vi "Potenza_celle.vi"() -> ()   [LabVIEW 2014]
uses:
  <vilib>/DAQmx/read.llb/DAQmx Read (Analog 2D DBL NChan NSamp).vi
  <vilib>/Analysis/baseanly.llb/Mean (DBL).vi
  <vilib>/DAQmx/create/channels.llb/DAQmx Create Channel (AI-Voltage-Basic).vi
  <vilib>/DAQmx/configure/timing.llb/DAQmx Timing (Sample Clock).vi
  <vilib>/DAQmx/miscellaneous.llb/DAQmx Fill In Error Info.vi
  <vilib>/Utility/file.llb/Write To Spreadsheet File (DBL).vi
  <vilib>/Analysis/NI_AALBase.lvlib
panel:
  in  "EXIT PROGRAM":bool
  in  "Resistenza":dbl=2.7 max=100000.0
  out "V_in(Volt)":dbl=0.2081706318888552 format="%.3f"
  out "Corrente (mA)":dbl=31.30588570078624 format="%.4f"
  in  "Fondo Scala AI1":dbl(ring)=5.0 items=["10"=10.0, "5"=5.0, "0.5"=0.5, "0.05"=0.05]
  in  "Fondo Scala AI0":dbl(ring)=0.5 items=["10"=10.0, "5"=5.0, "0.5"=0.5, "0.05"=0.05]
  in  "SALVA":bool=TRUE caption="ON\nOFF"
  out "power":cluster{dbl[], dbl[]}(graph)={[0.09478601789846895, 0.09478601789846895, 0.09519039454598441, 0.09519039454598441, 0.3692276546350666, 0.4111200013938477, 0.4111200013938477, 0.4208531577637632, 0.4208531577637632, 0.4255494982926404, 0.4402842388163407, 0.4435502862815671, 0.4435502862815671, 0.44368850953661537, 0.4491531483812087, 0.4513869200218114, 0.4513869200218114, 0.45480397968233355, 0.45480397968233355, 0.45705907451385963, 0.4584212187749075, 0.4605463340716431, 0.4605463340716431, 0.46217820728083553, 0.46357193005389463, 0.46446569248379926, 0.46484304010372907, 0.46543718331130957, 0.46615517263540734, 0.4390290005440171, 0.4390290005440171, 0.43334036436093054, 0.43334036436093054, 0.42420559561340954, 0.42420559561340954, 0.4270359081737125, 0.4270359081737125, 0.09544674857174822, 0.37267076173351704, 0.3881547056875887, 0.3881547056875887, 0.34106855480092135, 0.34106855480092135, 0.33109283770712306, 0.2068409232584436, 0.10409528201129736, 0.13447294260520917, 0.2984566947389119, 0.2984566947389119, 0.3700736078553747, 0.30440398953826114, 0.28259027086581395, 0.28259027086581395, 0.20417926683366502, 0.11794074102482587, 0.09686599380581434, 0.09553963187698407, 0.14140615930871372, 0.1509254439913714, 0.17778242825196688, 0.21380625131901929, 0.23492205647612335, 0.23492205647612335, 0.2729712800826533, 0.0, 0.0, 0.0, 0.0, 0.0, 0.0, 0.0, 0.0, 0.0, 0.0, 0.0, 0.0, 0.0, 0.0, 0.0, 0.0, 0.0, 0.0, 0.0, 0.0, 0.0, 0.0, 0.0, 0.0, 0.0, 0.0, 0.0, 0.0, 0.0, 0.0, 0.0, 0.0, 0.0, 0.0, 0.0, 0.0, 0.0, 0.0, 0.0, 0.0, 0.0, 0.0, 0.0, 0.0, 0.0, 0.0, 0.0, 0.0, 0.0, 0.0, 0.0, 0.0, 0.0, 0.0, 0.0, 0.0, 0.0, 0.0, 0.0, 0.0, 0.0, 0.0, 0.0, 0.0, 0.0, 0.0, 0.0, 0.0, 0.0, 0.0, 0.0, 0.0, 0.0, 0.0, 0.0, 0.0, 0.0, 0.0, 0.0, 0.0, 0.0, 0.0, 0.0, 0.0, 0.0, 0.0, 0.0, 0.0, 0.0, 0.0, 0.0, 0.0, 0.0, 0.0, 0.0, 0.0, 0.0, 0.0, 0.0, 0.0, 0.0, 0.0, 0.0, 0.0, 0.0, 0.0, 0.0, 0.0, 0.0, 0.0, 0.0, 0.0, 0.0, 0.0, 0.0, 0.0, 0.0, 0.0, 0.0, 0.0, 0.0, 0.0, 0.0, 0.0, 0.0, 0.0, 0.0, 0.0, 0.0, 0.0, 0.0, 0.0, 0.0, 0.0, 0.0, 0.0], [3.0170134735409397, 3.0170134735409397, 3.0201788565517984, 3.0201788565517984, 9.14140352368766, 7.85175000034162, 7.85175000034162, 7.221469220246045, 7.221469220246045, 6.8646837395680755, 5.412997641292046, 5.0489168328723055, 5.0489168328723055, 5.051448234534376, 4.348133054214019, 4.029529214267265, 4.029529214267265, 3.5183173733443494, 3.5183173733443494, 3.171630872751192, 2.9635146740029863, 2.588907716393703, 2.588907716393703, 2.2923528624342913, 2.0225602902113007, 1.8499819150481303, 1.7847675230358468, 1.6363589222375279, 1.534204978184801, 5.469082937412574, 5.469082937412574, 6.034056487177778, 6.034056487177778, 6.828298799638558, 6.828298799638558, 6.584690682350574, 6.584690682350574, 3.0455608576711226, 8.999642211687378, 8.636150436075797, 8.636150436075797, 9.145710007035497, 9.145710007035497, 9.095897977030202, 6.401982512490315, 3.325324661201692, 4.279414951081421, 8.728058986798336, 8.728058986798336, 9.110541910816105, 8.810402080562293, 8.426688585183642, 8.426688585183642, 6.40651230214226, 3.7818575624102304, 3.1124825241913823, 3.07055743646646, 4.5111823216029405, 4.79808672222816, 5.612649488498093, 6.681955401946596, 7.264660979738571, 7.264660979738571, 8.215200355082505, 0.0, 0.0, 0.0, 0.0, 0.0, 0.0, 0.0, 0.0, 0.0, 0.0, 0.0, 0.0, 0.0, 0.0, 0.0, 0.0, 0.0, 0.0, 0.0, 0.0, 0.0, 0.0, 0.0, 0.0, 0.0, 0.0, 0.0, 0.0, 0.0, 0.0, 0.0, 0.0, 0.0, 0.0, 0.0, 0.0, 0.0, 0.0, 0.0, 0.0, 0.0, 0.0, 0.0, 0.0, 0.0, 0.0, 0.0, 0.0, 0.0, 0.0, 0.0, 0.0, 0.0, 0.0, 0.0, 0.0, 0.0, 0.0, 0.0, 0.0, 0.0, 0.0, 0.0, 0.0, 0.0, 0.0, 0.0, 0.0, 0.0, 0.0, 0.0, 0.0, 0.0, 0.0, 0.0, 0.0, 0.0, 0.0, 0.0, 0.0, 0.0, 0.0, 0.0, 0.0, 0.0, 0.0, 0.0, 0.0, 0.0, 0.0, 0.0, 0.0, 0.0, 0.0, 0.0, 0.0, 0.0, 0.0, 0.0, 0.0, 0.0, 0.0, 0.0, 0.0, 0.0, 0.0, 0.0, 0.0, 0.0, 0.0, 0.0, 0.0, 0.0, 0.0, 0.0, 0.0, 0.0, 0.0, 0.0, 0.0, 0.0, 0.0, 0.0, 0.0, 0.0, 0.0, 0.0, 0.0, 0.0, 0.0, 0.0, 0.0, 0.0, 0.0, 0.0, 0.0]}
  out "Corrente":dbl[](array[numeric])=[31.82973122441588, 31.82973122441588, 31.727769077507247, 31.727769077507247, 24.758176720870885, 19.098438348222675, 19.098438348222675, 17.159118535828263, 17.159118535828263, 16.131340225073874, 12.294325265524694, 11.382963756373808, 11.382963756373808, 11.38512295441247, 9.680736002597579, 8.92699596628222, 8.92699596628222, 7.735898388140281, 7.735898388140281, 6.939214315183709, 6.464610608389228, 5.621383832339808, 5.621383832339808, 4.959889554120362, 4.3629912837392, 3.9830324284126934, 3.8395057450738177, 3.5157460145229575, 3.291189432718672, 12.457224763365586, 12.457224763365586, 13.92451980806476, 13.92451980806476, 16.096673099666933, 16.096673099666933, 15.41952457935226, 15.41952457935226, 31.90848198859017, 24.14904289734081, 22.249248326842938, 22.249248326842938, 26.814873075513415, 26.814873075513415, 27.472348964178497, 30.951237364625207, 31.945008428343538, 31.823613495579487, 29.24397120471226, 29.24397120471226, 24.618188699304703, 28.943122900348506, 29.81945754666479, 29.81945754666479, 31.37689933699946, 32.06574360605527, 32.13183906863047, 32.13909637437248, 31.902304281910812, 31.79110556403248, 31.57032752721442, 31.252385562742422, 30.923707585017354, 30.923707585017354, 30.095475071938026] format="%#_3f"
  out "Tensione":dbl[](array[numeric])=[0.09478601789846895, 0.09478601789846895, 0.09519039454598441, 0.09519039454598441, 0.3692276546350666, 0.4111200013938477, 0.4111200013938477, 0.4208531577637632, 0.4208531577637632, 0.4255494982926404, 0.4402842388163407, 0.4435502862815671, 0.4435502862815671, 0.44368850953661537, 0.4491531483812087, 0.4513869200218114, 0.4513869200218114, 0.45480397968233355, 0.45480397968233355, 0.45705907451385963, 0.4584212187749075, 0.4605463340716431, 0.4605463340716431, 0.46217820728083553, 0.46357193005389463, 0.46446569248379926, 0.46484304010372907, 0.46543718331130957, 0.46615517263540734, 0.4390290005440171, 0.4390290005440171, 0.43334036436093054, 0.43334036436093054, 0.42420559561340954, 0.42420559561340954, 0.4270359081737125, 0.4270359081737125, 0.09544674857174822, 0.37267076173351704, 0.3881547056875887, 0.3881547056875887, 0.34106855480092135, 0.34106855480092135, 0.33109283770712306, 0.2068409232584436, 0.10409528201129736, 0.13447294260520917, 0.2984566947389119, 0.2984566947389119, 0.3700736078553747, 0.30440398953826114, 0.28259027086581395, 0.28259027086581395, 0.20417926683366502, 0.11794074102482587, 0.09686599380581434, 0.09553963187698407, 0.14140615930871372, 0.1509254439913714, 0.17778242825196688, 0.21380625131901929, 0.23492205647612335, 0.23492205647612335, 0.2729712800826533] format="%#_3f"
  out "Potenza (mW)":dbl[](array[numeric])=[3.0170134735409397, 3.0170134735409397, 3.0201788565517984, 3.0201788565517984, 9.14140352368766, 7.85175000034162, 7.85175000034162, 7.221469220246045, 7.221469220246045, 6.8646837395680755, 5.412997641292046, 5.0489168328723055, 5.0489168328723055, 5.051448234534376, 4.348133054214019, 4.029529214267265, 4.029529214267265, 3.5183173733443494, 3.5183173733443494, 3.171630872751192, 2.9635146740029863, 2.588907716393703, 2.588907716393703, 2.2923528624342913, 2.0225602902113007, 1.8499819150481303, 1.7847675230358468, 1.6363589222375279, 1.534204978184801, 5.469082937412574, 5.469082937412574, 6.034056487177778, 6.034056487177778, 6.828298799638558, 6.828298799638558, 6.584690682350574, 6.584690682350574, 3.0455608576711226, 8.999642211687378, 8.636150436075797, 8.636150436075797, 9.145710007035497, 9.145710007035497, 9.095897977030202, 6.401982512490315, 3.325324661201692, 4.279414951081421, 8.728058986798336, 8.728058986798336, 9.110541910816105, 8.810402080562293, 8.426688585183642, 8.426688585183642, 6.40651230214226, 3.7818575624102304, 3.1124825241913823, 3.07055743646646, 4.5111823216029405, 4.79808672222816, 5.612649488498093, 6.681955401946596, 7.264660979738571, 7.264660979738571, 8.215200355082505] format="%#_3f"
  out "Grafico Dati Acquisiti":cluster{dbl[], dbl[]}(graph)={[0.09478601789846895, 0.09478601789846895, 0.09519039454598441, 0.09519039454598441, 0.3692276546350666, 0.4111200013938477, 0.4111200013938477, 0.4208531577637632, 0.4208531577637632, 0.4255494982926404, 0.4402842388163407, 0.4435502862815671, 0.4435502862815671, 0.44368850953661537, 0.4491531483812087, 0.4513869200218114, 0.4513869200218114, 0.45480397968233355, 0.45480397968233355, 0.45705907451385963, 0.4584212187749075, 0.4605463340716431, 0.4605463340716431, 0.46217820728083553, 0.46357193005389463, 0.46446569248379926, 0.46484304010372907, 0.46543718331130957, 0.46615517263540734, 0.4390290005440171, 0.4390290005440171, 0.43334036436093054, 0.43334036436093054, 0.42420559561340954, 0.42420559561340954, 0.4270359081737125, 0.4270359081737125, 0.09544674857174822, 0.37267076173351704, 0.3881547056875887, 0.3881547056875887, 0.34106855480092135, 0.34106855480092135, 0.33109283770712306, 0.2068409232584436, 0.10409528201129736, 0.13447294260520917, 0.2984566947389119, 0.2984566947389119, 0.3700736078553747, 0.30440398953826114, 0.28259027086581395, 0.28259027086581395, 0.20417926683366502, 0.11794074102482587, 0.09686599380581434, 0.09553963187698407, 0.14140615930871372, 0.1509254439913714, 0.17778242825196688, 0.21380625131901929, 0.23492205647612335, 0.23492205647612335, 0.2729712800826533, 0.0, 0.0, 0.0, 0.0, 0.0, 0.0, 0.0, 0.0, 0.0, 0.0, 0.0, 0.0, 0.0, 0.0, 0.0, 0.0, 0.0, 0.0, 0.0, 0.0, 0.0, 0.0, 0.0, 0.0, 0.0, 0.0, 0.0, 0.0, 0.0, 0.0, 0.0, 0.0, 0.0, 0.0, 0.0, 0.0, 0.0, 0.0, 0.0, 0.0, 0.0, 0.0, 0.0, 0.0, 0.0, 0.0, 0.0, 0.0, 0.0, 0.0, 0.0, 0.0, 0.0, 0.0, 0.0, 0.0, 0.0, 0.0, 0.0, 0.0, 0.0, 0.0, 0.0, 0.0, 0.0, 0.0, 0.0, 0.0, 0.0, 0.0, 0.0, 0.0, 0.0, 0.0, 0.0, 0.0, 0.0, 0.0, 0.0, 0.0, 0.0, 0.0, 0.0, 0.0, 0.0, 0.0, 0.0, 0.0, 0.0, 0.0, 0.0, 0.0, 0.0, 0.0, 0.0, 0.0, 0.0, 0.0, 0.0, 0.0, 0.0, 0.0, 0.0, 0.0, 0.0, 0.0, 0.0, 0.0, 0.0, 0.0, 0.0, 0.0, 0.0, 0.0, 0.0, 0.0, 0.0, 0.0, 0.0, 0.0, 0.0, 0.0, 0.0, 0.0, 0.0, 0.0, 0.0, 0.0, 0.0, 0.0, 0.0, 0.0, 0.0, 0.0, 0.0, 0.0], [31.82973122441588, 31.82973122441588, 31.727769077507247, 31.727769077507247, 24.758176720870885, 19.098438348222675, 19.098438348222675, 17.159118535828263, 17.159118535828263, 16.131340225073874, 12.294325265524694, 11.382963756373808, 11.382963756373808, 11.38512295441247, 9.680736002597579, 8.92699596628222, 8.92699596628222, 7.735898388140281, 7.735898388140281, 6.939214315183709, 6.464610608389228, 5.621383832339808, 5.621383832339808, 4.959889554120362, 4.3629912837392, 3.9830324284126934, 3.8395057450738177, 3.5157460145229575, 3.291189432718672, 12.457224763365586, 12.457224763365586, 13.92451980806476, 13.92451980806476, 16.096673099666933, 16.096673099666933, 15.41952457935226, 15.41952457935226, 31.90848198859017, 24.14904289734081, 22.249248326842938, 22.249248326842938, 26.814873075513415, 26.814873075513415, 27.472348964178497, 30.951237364625207, 31.945008428343538, 31.823613495579487, 29.24397120471226, 29.24397120471226, 24.618188699304703, 28.943122900348506, 29.81945754666479, 29.81945754666479, 31.37689933699946, 32.06574360605527, 32.13183906863047, 32.13909637437248, 31.902304281910812, 31.79110556403248, 31.57032752721442, 31.252385562742422, 30.923707585017354, 30.923707585017354, 30.095475071938026, 0.0, 0.0, 0.0, 0.0, 0.0, 0.0, 0.0, 0.0, 0.0, 0.0, 0.0, 0.0, 0.0, 0.0, 0.0, 0.0, 0.0, 0.0, 0.0, 0.0, 0.0, 0.0, 0.0, 0.0, 0.0, 0.0, 0.0, 0.0, 0.0, 0.0, 0.0, 0.0, 0.0, 0.0, 0.0, 0.0, 0.0, 0.0, 0.0, 0.0, 0.0, 0.0, 0.0, 0.0, 0.0, 0.0, 0.0, 0.0, 0.0, 0.0, 0.0, 0.0, 0.0, 0.0, 0.0, 0.0, 0.0, 0.0, 0.0, 0.0, 0.0, 0.0, 0.0, 0.0, 0.0, 0.0, 0.0, 0.0, 0.0, 0.0, 0.0, 0.0, 0.0, 0.0, 0.0, 0.0, 0.0, 0.0, 0.0, 0.0, 0.0, 0.0, 0.0, 0.0, 0.0, 0.0, 0.0, 0.0, 0.0, 0.0, 0.0, 0.0, 0.0, 0.0, 0.0, 0.0, 0.0, 0.0, 0.0, 0.0, 0.0, 0.0, 0.0, 0.0, 0.0, 0.0, 0.0, 0.0, 0.0, 0.0, 0.0, 0.0, 0.0, 0.0, 0.0, 0.0, 0.0, 0.0, 0.0, 0.0, 0.0, 0.0, 0.0, 0.0, 0.0, 0.0, 0.0, 0.0, 0.0, 0.0, 0.0, 0.0, 0.0, 0.0, 0.0, 0.0]}
  out "Pronto per la misura":bool=TRUE
  in  "Esegui la misura":bool
  out "Misure fatte":u16=64
  # "Dati acquisiti"
  # "NO\nSI"
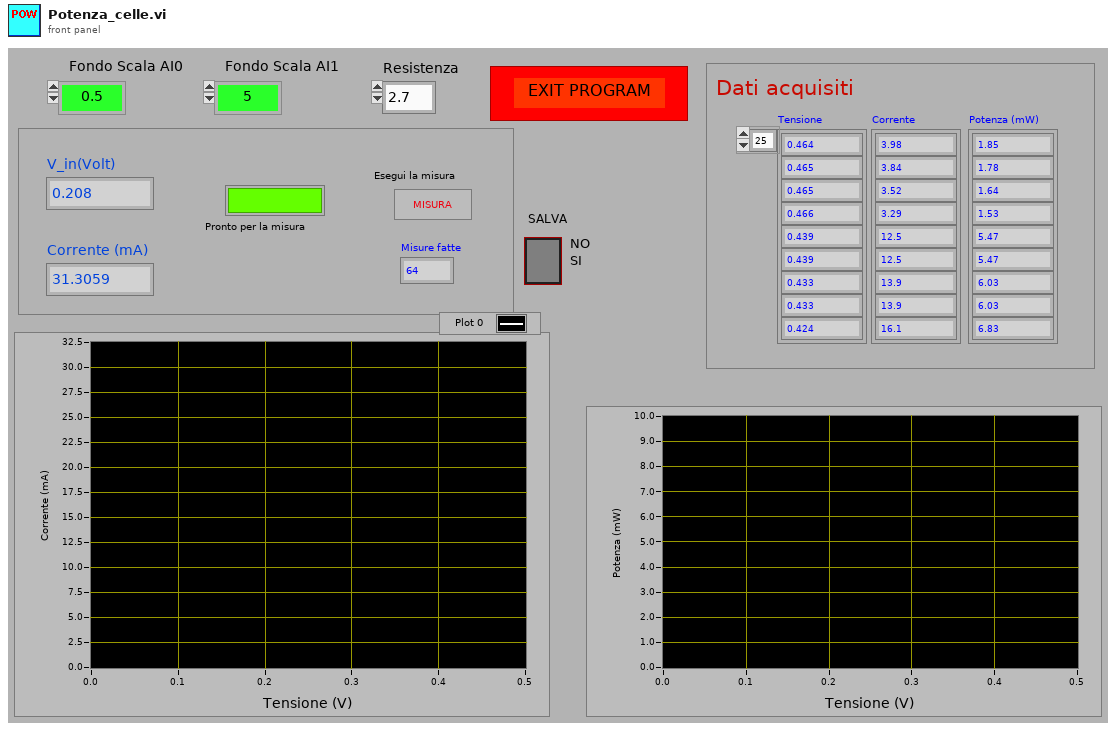
[diagram p1: front panel]
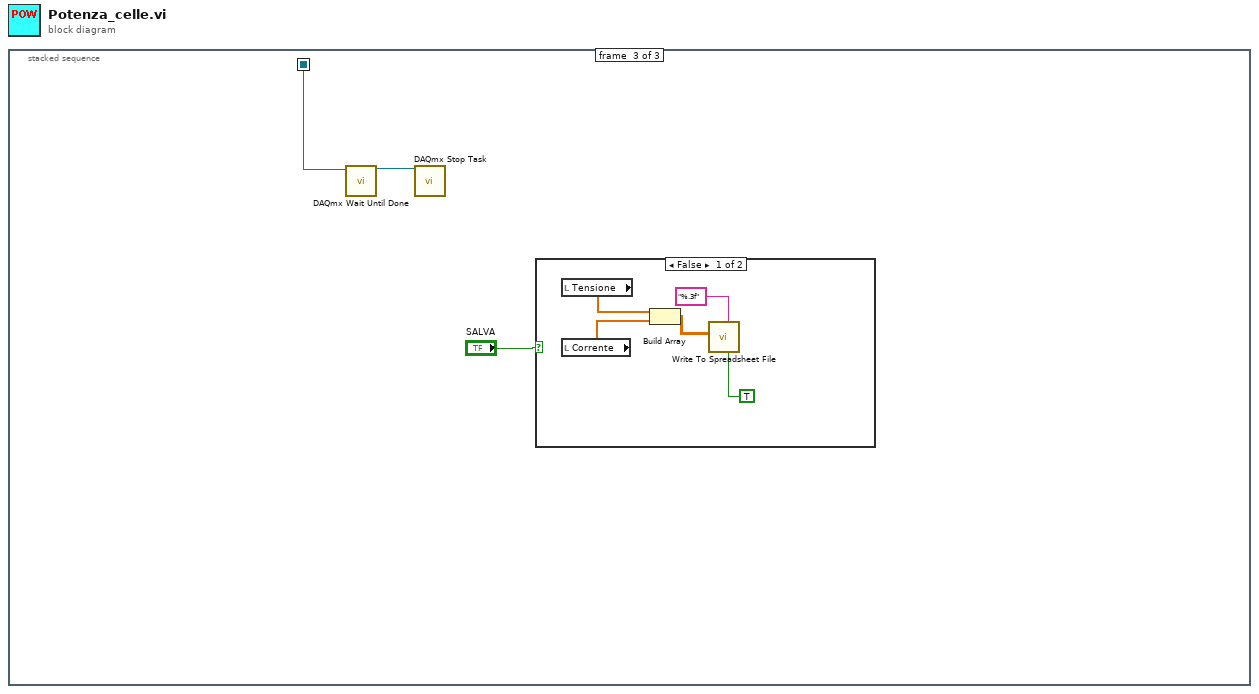
[diagram p0: block diagram]
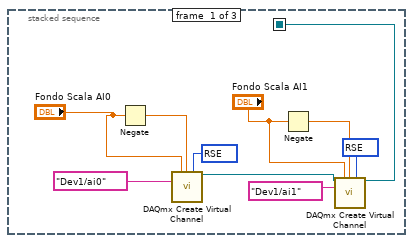
[diagram p2: hidden frame]
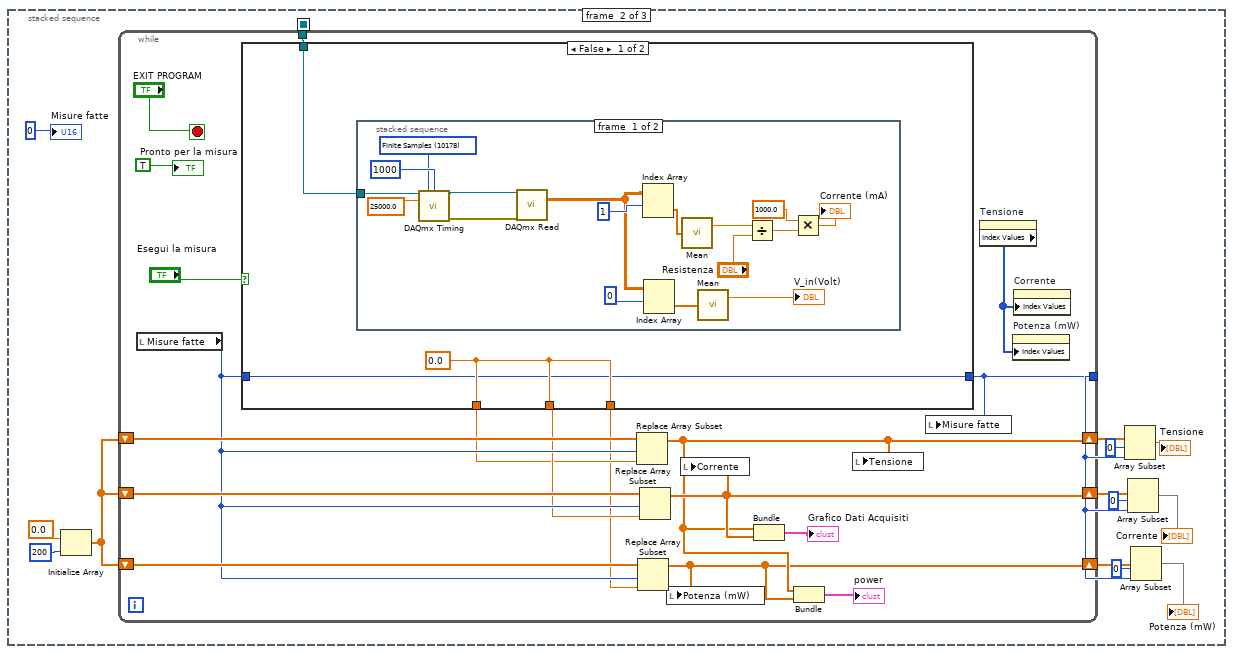
[diagram p3: hidden frame]
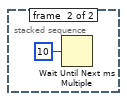
[diagram p4: hidden frame]
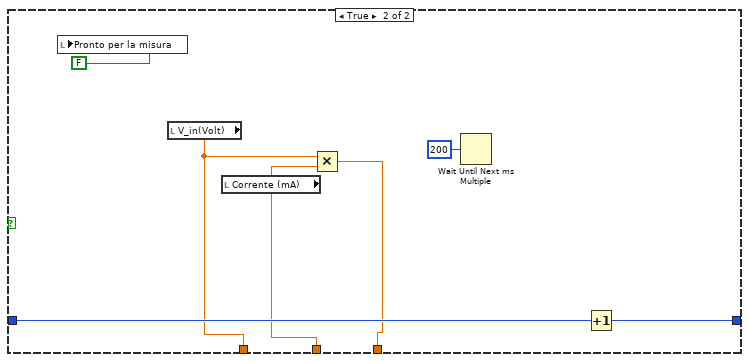
[diagram p5: hidden frame]
diagram:
  n1 = stacked-sequence {
    seq-local: [w1 _ _] -> [_ w11 w72]
    frame #0 {
      w6 = 10083 items=["default"=-1, "RSE"=10083, "NRSE"=10078, "Differential"=10106, "Pseudodifferential"=12529] ("input terminal configuration")
      w9 = 10083 items=["default"=-1, "RSE"=10083, "NRSE"=10078, "Differential"=10106, "Pseudodifferential"=12529] ("input terminal configuration")
      n2 = Negate(x="Fondo Scala AI0") -> (-x=w7:dbl)
      n3 = call-poly <vilib>:"DAQmx Create Virtual Channel.vi"("maximum value"="Fondo Scala AI0", "minimum value"=w7, "input terminal configuration"=w6, "physical channels"=tag "Dev1/ai0") -> ("task out"=w4:refnum<k21>)  [unwired: 5 in, 6 out]
      n4 = Negate(x="Fondo Scala AI1") -> (-x=w10:dbl)
      n5 = call-poly <vilib>:"DAQmx Create Virtual Channel.vi"("task in"=w4, "maximum value"="Fondo Scala AI1", "minimum value"=w10, "input terminal configuration"=w9, "physical channels"=tag "Dev1/ai1") -> ("task out"=w1:refnum<k21>)  [unwired: 4 in, 6 out]
    }
    frame #1 {
      n6 = Initialize Array(0.0 ("Element Data"), 200 ("Dimension Size")) -> (w22:dbl[])
      n7 = while {
        tunnel: [w41] -> w15
        shift-left: w22 -> [w38]
        shift-right: [w32] -> w18
        shift-left: w22 -> [w39]
        shift-right: [w30] -> w21
        shift-left: w22 -> [w40]
        shift-right: [w29] -> w16
        tunnel: w11 -> [w28]
        stop <- "EXIT PROGRAM" stop-if-true
        n8 = local read "Misure fatte"() -> (w37:u16)
        n9 = case shown="False" "Esegui la misura" {
          tunnel: w37 -> [w44 w71]
          tunnel: [w44 w65] -> w41
          tunnel: [w45 w68] -> w35
          tunnel: [w45 w67] -> w36
          tunnel: [w45 w66] -> w34
          tunnel: w28 -> [w46 _]
          frame False {
            w45 = 0.0
            n10 = stacked-sequence {
              tunnel: w46 -> [w58 _]
              frame #0 {
                w59 = 10178 items=["Finite Samples"=10178, "Continuous Samples"=10123, "Hardware Timed Single Point"=12522] ("sample mode")
                n11 = call-poly <vilib>:"DAQmx Timing.vi"("task/channels in"=w58, "sample mode"=w59, "samples per channel"=u32 1000, "rate"=25000.0) -> ("task out"=w63:refnum<k21>, "error out"=w62:errorcluster)  [unwired: 3 in, 7 out]
                n12 = call-poly <vilib>:"DAQmx Read.vi"("task/channels in"=w63, "error in"=w62) -> ("data"=w47:dbl[][])  [unwired: 1 in, 12 out]
                n13 = Index Array(array=w47, index (row)=1) -> (element=w55:dbl[])  [unwired: 1 in]
                n14 = Index Array(array=w47, index (row)=0) -> (element=w54:dbl[])  [unwired: 1 in]
                n15 = call-poly <vilib>:"Mean.vi"("X"=w55) -> ("mean"=w57:dbl)  [unwired: 1 out]
                n16 = call-poly <vilib>:"Mean.vi"("X"=w54) -> ("mean"=→"V_in(Volt)":dbl)  [unwired: 1 out]
                n17 = Divide(x=w57, y="Resistenza") -> (x/y=w51:dbl)
                n18 = Multiply(x=1000.0, y=w51) -> (x*y=→"Corrente (mA)":dbl)
              }
              frame #1 {
                n19 = Wait Until Next ms Multiple(millisecond multiple=u32 10) -> ()  [unwired: 1 out]
              }
            }
          }
          frame True {
            n20 = local write "Pronto per la misura"(FALSE ("Pronto per la misura")) -> ()
            n21 = local read "V_in(Volt)"() -> (w68:dbl)
            n22 = local read "Corrente (mA)"() -> (w67:dbl)
            n23 = Multiply(x=w68, y=w67) -> (x*y=w66:dbl)
            n24 = Wait Until Next ms Multiple(millisecond multiple=u32 200) -> ()  [unwired: 1 out]
            n25 = Increment(x=w71) -> (x+1=w65:u16)
          }
        }
        n26 = Replace Array Subset(array=w39, new element=w35, index=w37) -> (w30:dbl[])
        n27 = Replace Array Subset(array=w40, new element=w34, index=w37) -> (w29:dbl[])
        n28 = Replace Array Subset(array=w38, new element=w36, index=w37) -> (w32:dbl[])
        n29 = local write "Potenza (mW)"(w29) -> ()
        n30 = local write "Corrente"(w32) -> ()
        n31 = Bundle(w30, w32) -> (→"Grafico Dati Acquisiti":cluster{dbl[], dbl[]})  [unwired: 1 out]
        n32 = Bundle(w30, w29) -> (→"power":cluster{dbl[], dbl[]})  [unwired: 1 out]
        n33 = local write "Tensione"(w30) -> ()
        n34 = local write "Misure fatte"(w41) -> ()
        n35 = property on="Tensione" class="Arr (strict)"() -> ("Index Values"=w27:u32[])  [unwired: 2 in, 2 out]
        n36 = property on="Potenza (mW)" class="Arr (strict)"("Index Values"=w27) -> ()  [unwired: 2 in, 2 out]
        n37 = property on="Corrente" class="Arr (strict)"("Index Values"=w27) -> ()  [unwired: 2 in, 2 out]
        "Pronto per la misura" <- TRUE ("Pronto per la misura")
      }
      n38 = Array Subset(array=w21, index=0 ("Array Index"), length=w15) -> (→"Tensione":dbl[])
      n39 = Array Subset(array=w18, index=0 ("Array Index"), length=w15) -> (→"Corrente":dbl[])
      n40 = Array Subset(array=w16, index=0 ("Array Index"), length=w15) -> (→"Potenza (mW)":dbl[])
      "Misure fatte" <- u16 0
    }
    frame #2 {
      n41 = call <vilib>:"DAQmx Wait Until Done.vi"("task/channels in"=w72) -> ("task out"=w73:refnum<k21>)  [unwired: 2 in, 12 out]
      n42 = call <vilib>:"DAQmx Stop Task.vi"("task/channels in"=w73) -> ()  [unwired: 1 in, 14 out]
      n43 = case shown="False" "SALVA" {
        frame False {
          n44 = local read "Tensione"() -> (w76:dbl[])
          n45 = local read "Corrente"() -> (w75:dbl[])
          n46 = Build Array(w76, w75) -> (w79:dbl[][])
          n47 = call-poly <vilib>:"Write To Spreadsheet File.vi"("transpose? (no:F)"=TRUE, "format (%.3f)"="%.3f", "2D data"=w79) -> ()  [unwired: 3 in, 3 out]
        }
        frame True {
        }
      }
    }
  }
